vi "temp.vi"() -> ()   [LabVIEW 2011]
panel:
  out "二维图片 2":picture
  out "二维图片":picture
  in  "Integer":i32=1234
  in  "Fixpoint":fxp<+,10,11>=1234.0
  in  "Complex":cdb=1234.0+0.0i
  in  "Path":path
  in  "Class":refnum<class>
  in  "Error":errorcluster
  in  "簇":cluster{"String":string, "布尔":bool}={"String"="ABC", "布尔"=TRUE}
  in  "Number Cluster":cluster{"Float":dbl, "Integer":i32}={"Float"=12.34, "Integer"=1234}
  in  "String Array":string[](array[string])=["ABC"]
  in  "WaveForm":waveform(dbl)
  in  "String":string="ABC"
  in  "Float Array":dbl[](array[numeric])=[12.34]
  in  "TimeStamp":timestamp
  in  "Integer Array":i32[](array[numeric])=[1234, 5678]
  in  "Float":dbl=12.34
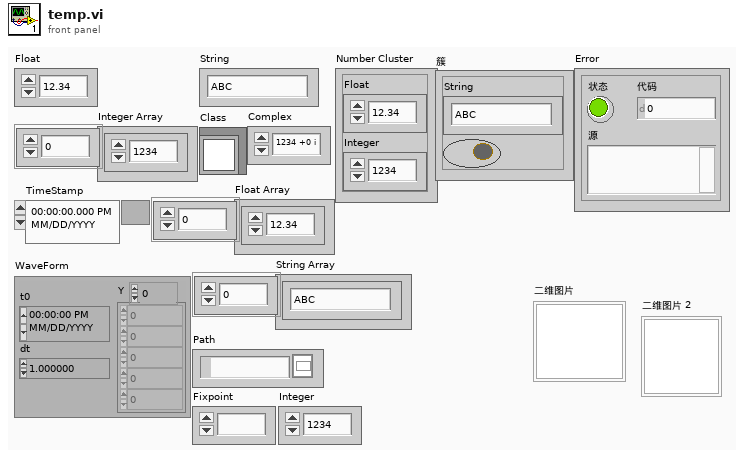
[diagram p1: front panel]
types:
  T1 = typedef "imagedata.ctl" = cluster{"image type":i32, "image depth":i32, "image":u8[], "mask":u8[], "colors":u32[], "Rectangle":cluster{"left":i16, "top":i16, "right":i16, "bottom":i16}}
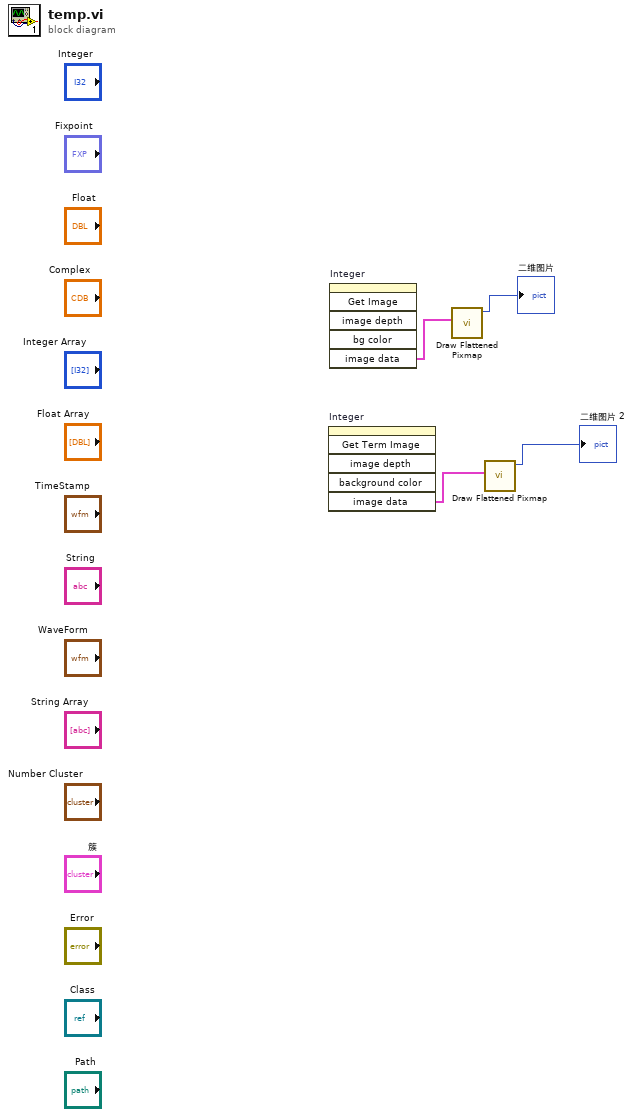
[diagram p0: block diagram]
diagram:
  n1 = invoke on="Integer" class="DigNum (严格)" method="Get Term Image"() -> ("image data"=w2:T1)  [unwired: 6 in, 5 out]
  n2 = invoke on="Integer" class="DigNum (严格)" method="Get Image"() -> ("image data"=w4:T1)  [unwired: 6 in, 5 out]
  n3 = call <vilib>:"Draw Flattened Pixmap.vi"("image data"=w4) -> ("new picture"=→"二维图片":picture)  [unwired: 8 in]
  n4 = call <vilib>:"Draw Flattened Pixmap.vi"("image data"=w2) -> ("new picture"=→"二维图片 2":picture)  [unwired: 8 in]
